vi "Apply Configuration.vi"(8 "error in (no error)":errorcluster, 11 "Thermometer Base in":refnum<class "Thermometer Base.lvclass">) -> (0 "error out":errorcluster, 3 "Thermometer Base out":refnum<class "Thermometer Base.lvclass">)   [LabVIEW 2023, in "Thermometer.lvlib" / "Thermometer Base.lvlib" / "Thermometer Base.lvclass"]
uses:
  Thermometer Base.lvclass
  Thermometer Base.lvclass/Thermometer Base.ctl
  Interfaces/IConfigure/IConfigure.lvclass
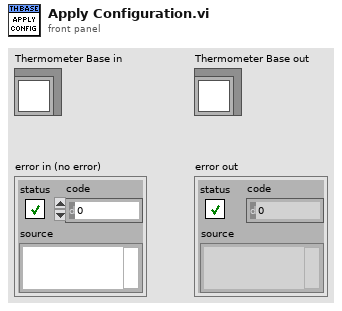
[diagram p1: front panel]
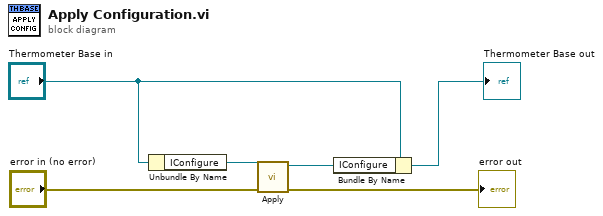
[diagram p0: block diagram]
diagram:
  n1 = Unbundle By Name("Thermometer Base in") -> ("IConfigure"=w6:refnum<class "IConfigure.lvclass">)
  n2 = call-dynamic "Apply.vi"("Error In"="error in (no error)", "IConfigure in"=w6) -> ("Error Out"=→"error out":errorcluster, "IConfigure out"=w5:refnum<class "IConfigure.lvclass">)  [unwired: 8 in]
  n3 = Bundle By Name(cluster="Thermometer Base in", "IConfigure"=w5) -> (→"Thermometer Base out":refnum<class "Thermometer Base.lvclass">)
